vi "calc_scanner_pos.vi"(8 "error in (no error)":errorcluster, 11 "Mouse position":cluster{"X":i32, "Y":i32}) -> (0 "error out":errorcluster, 3 "Scanner position":dbl[](array[numeric]))   [LabVIEW 2011]
uses:
  global_image_size.vi
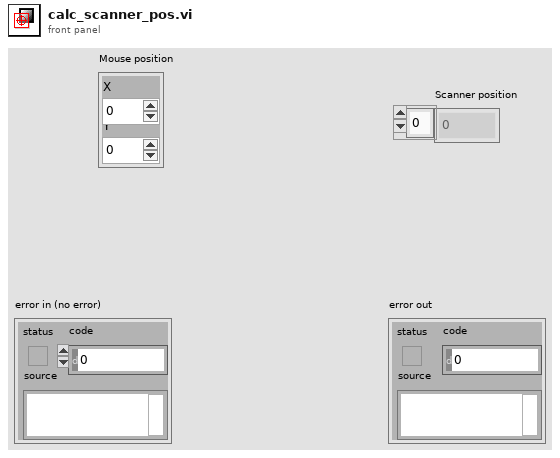
[diagram p1: front panel]
types:
  T1 = typedef "LVBoundsTypeDef.ctl" = cluster{"Width":u32, "Height":u32}
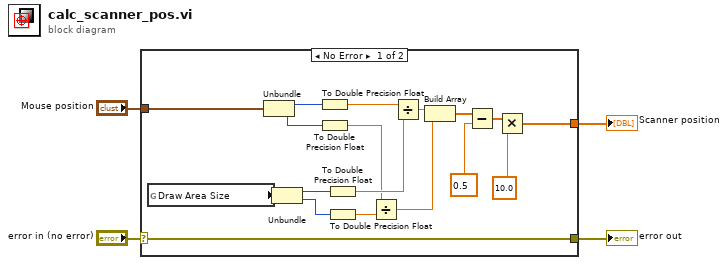
[diagram p0: block diagram]
diagram:
  n1 = case shown="No Error" "error in (no error)" {
    selector: "error in (no error)" -> [w22 w23]
    tunnel: [w22 w23] -> w3
    tunnel: "Mouse position" -> [w21 _]
    tunnel: [w5 _] -> w1
    frame No Error {
      n2 = global read "global_image_size.vi" "Draw Area Size"() -> (w10:T1)
      n3 = Unbundle(w21) -> ("X"=w18:i32, "Y"=w17:i32)
      n4 = Unbundle(w10) -> ("Width"=w20:u32, "Height"=w19:u32)
      n5 = To Double Precision Float(number=w18) -> (double precision float=w16:dbl)
      n6 = To Double Precision Float(number=w17) -> (double precision float=w14:dbl)
      n7 = To Double Precision Float(number=w20) -> (double precision float=w15:dbl)
      n8 = To Double Precision Float(number=w19) -> (double precision float=w13:dbl)
      n9 = Divide(x=w14, y=w13) -> (x/y=w11:dbl)
      n10 = Divide(x=w16, y=w15) -> (x/y=w12:dbl)
      n11 = Build Array(w12, w11) -> (w9:dbl[])
      n12 = Subtract(x=w9, y=0.5) -> (x-y=w8:dbl[])
      n13 = Multiply(x=w8, y=10.0 ("Scalefactor")) -> (x*y=w5:dbl[])
    }
    frame Error {
    }
  }
  "error out" <- w3
  "Scanner position" <- w1
